vi "flatSecuence.vi"() -> ()   [LabVIEW 2020]
panel:
  out "Thermometer 4":u8(slide) scale=0.0..100.0
  out "Thermometer 3":u8(slide) scale=0.0..100.0
  out "Thermometer 2":u8(slide) scale=0.0..100.0
  out "Thermometer":u8(slide) scale=0.0..100.0
  # "Flat Secuence"
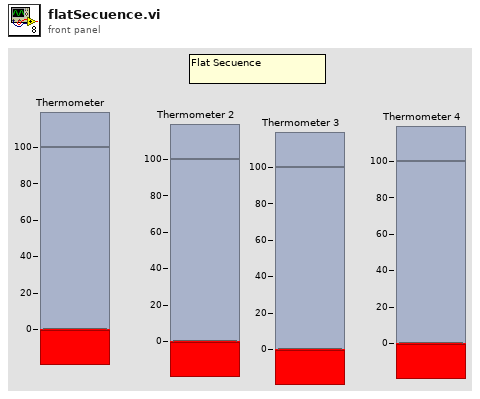
[diagram p1: front panel]
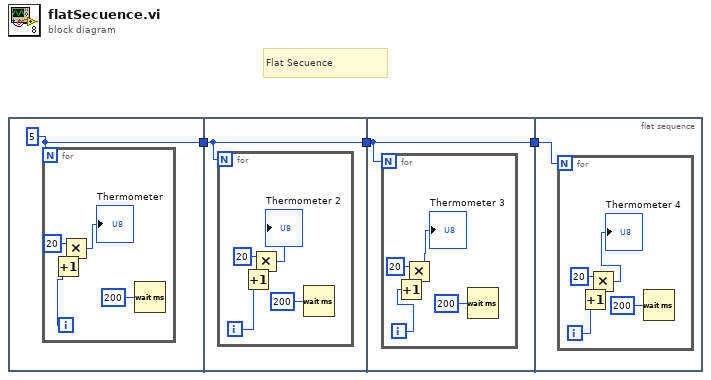
[diagram p0: block diagram]
diagram:
  # "Flat Secuence"
  n1 = flat-sequence {
    tunnel: [w4] -> w1
    tunnel: [w10] -> w2
    tunnel: w1 -> [w10]
    tunnel: [w16] -> w3
    tunnel: w2 -> [w16]
    tunnel: w3 -> [w22]
    frame #0 {
      w4 = 5
      n2 = for {
        N: w4 -> [_]
        i -> [w8]
        n3 = Increment(x=w8) -> (x+1=w6:i32)
        n4 = Multiply(x=20, y=w6) -> (x*y=→"Thermometer":i32)
        n5 = Wait (ms)(milliseconds to wait=u32 200) -> ()  [unwired: 1 out]
      }
    }
    frame #1 {
      n6 = for {
        N: w10 -> [_]
        i -> [w12]
        n7 = Increment(x=w12) -> (x+1=w14:i32)
        n8 = Multiply(x=20, y=w14) -> (x*y=→"Thermometer 2":i32)
        n9 = Wait (ms)(milliseconds to wait=u32 200) -> ()  [unwired: 1 out]
      }
    }
    frame #2 {
      n10 = for {
        N: w16 -> [_]
        i -> [w18]
        n11 = Increment(x=w18) -> (x+1=w20:i32)
        n12 = Multiply(x=20, y=w20) -> (x*y=→"Thermometer 3":i32)
        n13 = Wait (ms)(milliseconds to wait=u32 200) -> ()  [unwired: 1 out]
      }
    }
    frame #3 {
      n14 = for {
        N: w22 -> [_]
        i -> [w24]
        n15 = Increment(x=w24) -> (x+1=w26:i32)
        n16 = Multiply(x=20, y=w26) -> (x*y=→"Thermometer 4":i32)
        n17 = Wait (ms)(milliseconds to wait=u32 200) -> ()  [unwired: 1 out]
      }
    }
  }
